vi "Read Single Measurement.vi"   [LabVIEW 2012, in "MicroStrain 3DM-GXx.lvlib"]
doc: "Requests a single measurement and parse the return message from the device. This VI can only be used while the device is <B>not </B>in continuous measurement mode."
uses:
  <instrlib>/MicroStrain 3DM-GXx/MicroStrain 3DM-GXx.lvlib
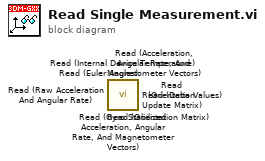
[diagram p0: block diagram]
diagram:
  n1 = call <instrlib>:"Read (Gyro Stabilized Acceleration, Angular Rate, And Magnetometer Vectors).vi"() -> ()  [unwired: 9 in, 7 out]
  n2 = call <instrlib>:"Read (Acceleration, Angular Rate, And Magnetometer Vectors).vi"() -> ()  [unwired: 9 in, 7 out]
  n3 = call <instrlib>:"Read (Raw Acceleration And Angular Rate).vi"() -> ()  [unwired: 10 in, 6 out]
  n4 = call <instrlib>:"Read (Delta Values).vi"() -> ()  [unwired: 10 in, 6 out]
  n5 = call <instrlib>:"Read (Euler Angles).vi"() -> ()  [unwired: 9 in, 7 out]
  n6 = call <instrlib>:"Read (Orientation Update Matrix).vi"() -> ()  [unwired: 11 in, 5 out]
  n7 = call <instrlib>:"Read (Orientation Matrix).vi"() -> ()  [unwired: 11 in, 5 out]
  n8 = call <instrlib>:"Read (Internal Device Temperature).vi"() -> ()  [unwired: 11 in, 5 out]
